vi "Full Channel ID.vi"(1 "Cluster":T2) -> (0 "String":string)   [LabVIEW 2017]
uses:
  Controls/Inst_type.ctl
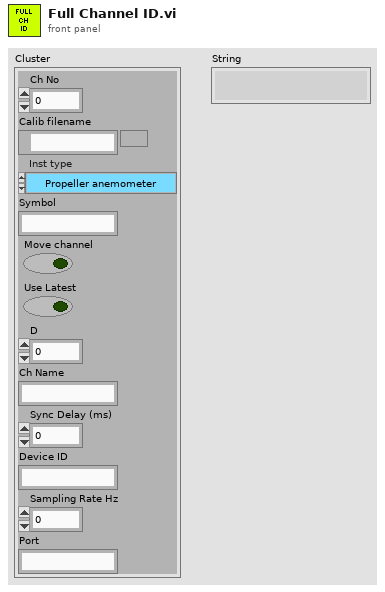
[diagram p1: front panel]
types:
  T1 = typedef "Inst_type.ctl" = enum16{"Propeller anemometer", "Raw voltage", "Pressure Transducer", "Pitot-static tube", "Preston tube", "Hot wire", "Cross wire 1", "Cross wire 2", "Generic Linear", "Generic Polynomial", "Generic BackPoly", "Fast FID", "Thermocouple", "Cold wire", "Pulsed Wire", "LDA Vel", "LDA Tran time", "LDA Arr time", "Microphone"}
  T2 = cluster{"Ch No":i16, "Calib filename":path, "Inst type":T1, "Symbol":string, "Move channel":bool, "Use Latest":bool, "D":dbl, "Ch Name":string, "Sync Delay (ms)":dbl, "Device ID":string, "Sampling Rate Hz":dbl, "Port":string}
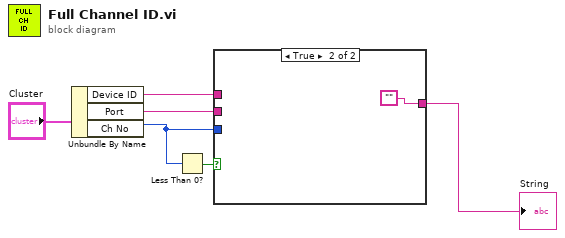
[diagram p0: block diagram]
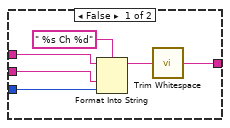
[diagram p2: hidden frame]
diagram:
  n1 = Unbundle By Name("Cluster") -> ("Device ID"=w5:string, "Port"=w4:string, "Ch No"=w2:i16)
  n2 = Less Than 0?(x=w2) -> (x < 0?=w1:bool)
  n3 = case shown="True" w1 {
    tunnel: w5 -> [w11 _]
    tunnel: w4 -> [w10 _]
    tunnel: [w8 ""] -> w3
    tunnel: w2 -> [w7 _]
    frame False {
      n4 = Format Into String(format string=" %s Ch %d", initial string=w11, w10, w7) -> (resulting string=w9:string)  [unwired: 1 in, 1 out]
      n5 = call <vilib>:"Trim Whitespace.vi"("string"=w9) -> ("trimmed string"=w8:string)  [unwired: 1 in]
    }
    frame True {
    }
  }
  "String" <- w3
